vi "process_control_handler.vi"(11 "Status Panel in":T1 {"Process Value" format="%#.3g"}) -> (3 "Status Panel out":T1 {"Process Value" format="%#.3g"})   [LabVIEW 2019]
uses:
  Week 4/Week 4 Student Material/Week 4 Student Material/Exercises 16/CLD 16 Status Panel.ctl
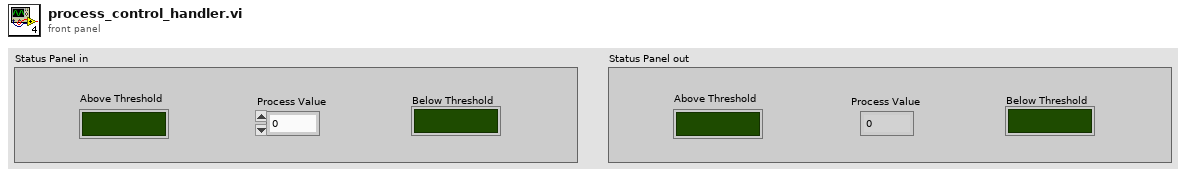
[diagram p1: front panel]
types:
  T1 = typedef "CLD 16 Status Panel.ctl" = cluster{"Above Threshold":bool, "Below Threshold":bool, "Process Value":dbl}
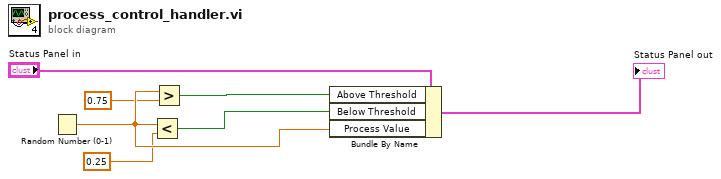
[diagram p0: block diagram]
diagram:
  n1 = Random Number (0-1)() -> (number: 0 to 1=w6:dbl)
  n2 = Less?(x=w6, y=0.25) -> (x < y?=w5:bool)
  n3 = Greater?(x=w6, y=0.75) -> (0:w4:bool)
  n4 = Bundle By Name(cluster="Status Panel in", "Above Threshold"=w4, "Below Threshold"=w5, "Process Value"=w6) -> (→"Status Panel out":T1)
